vi "Function_Eval.vi"() -> ()   [LabVIEW 2022 SP3]
panel:
  out "f(x, y)":dbl format="%.2f"
  in  "Y":dbl
  in  "X":dbl
  # "Function_Eval:\nIn the boxes below, enter any float value for both x and y.\nThe output will be the solution to the following function:\nf(x, y) = 4x^3 + 3y^2 + 7xy"
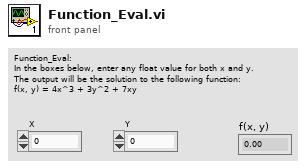
[diagram p1: front panel]
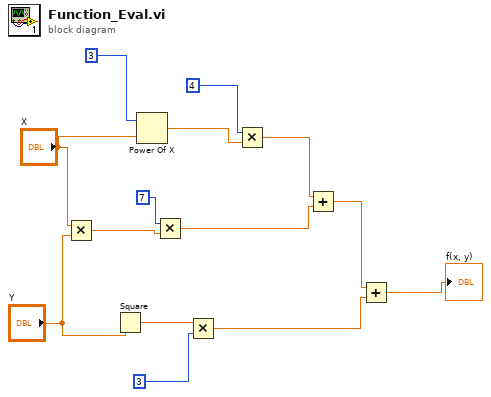
[diagram p0: block diagram]
diagram:
  n1 = Multiply(x="X", y="Y") -> (x*y=w7:dbl)
  n2 = Square(x="Y") -> (x^2=w11:dbl)
  n3 = Power Of X(1:"X", 2:3) -> (0:w13:dbl)
  n4 = Multiply(x=7, y=w7) -> (x*y=w6:dbl)
  n5 = Multiply(x=w11, y=3) -> (x*y=w3:dbl)
  n6 = Multiply(x=4, y=w13) -> (x*y=w5:dbl)
  n7 = Add(x=w5, y=w6) -> (x+y=w2:dbl)
  n8 = Add(x=w2, y=w3) -> (x+y=→"f(x, y)":dbl)
